vi "TXT_to_Pos_Array.vi"(11 "pointfile":path) -> (0 "errorString":string, 1 "pointIDs":string[](array[string]), 2 "pointComments":string[](array[string]), 3 "pointsXYZArray":dbl[][](array[numeric]), 4 "File Path Out":path, 5 "Number of Points":i32)   [LabVIEW 2021]
uses:
  <vilib>/Math Plots/3D Math Plots/3D Scatter/3D Scatter XCtrl/3D Scatter.xctl
  <vilib>/Math Plots/3D Math Plots/3D Plot/3D Plot Datatype/3D Plot Datatype.lvclass
  Globals/Trav_pos_global.vi
  <vilib>/Utility/file.llb/Read Delimited Spreadsheet (string).vi
  <vilib>/Math Plots/3D Math Plots/3D Scatter/3D Scatter Datatype/Public/Plot Helper (Vector).vi
  <vilib>/Math Plots/3D Math Plots/3D Scatter/3D Scatter Datatype/3D Scatter Datatype.lvclass
panel:
  out "fileRead":string[][](array[string])
  out "pointCloud":refnum<class "3D Plot Datatype.lvclass">[](xcontrol)
  # "If relative path given, prepended with path to MR file"
  # "Expects 4-row header!"
  # "Sometimes this indicator disappears..."
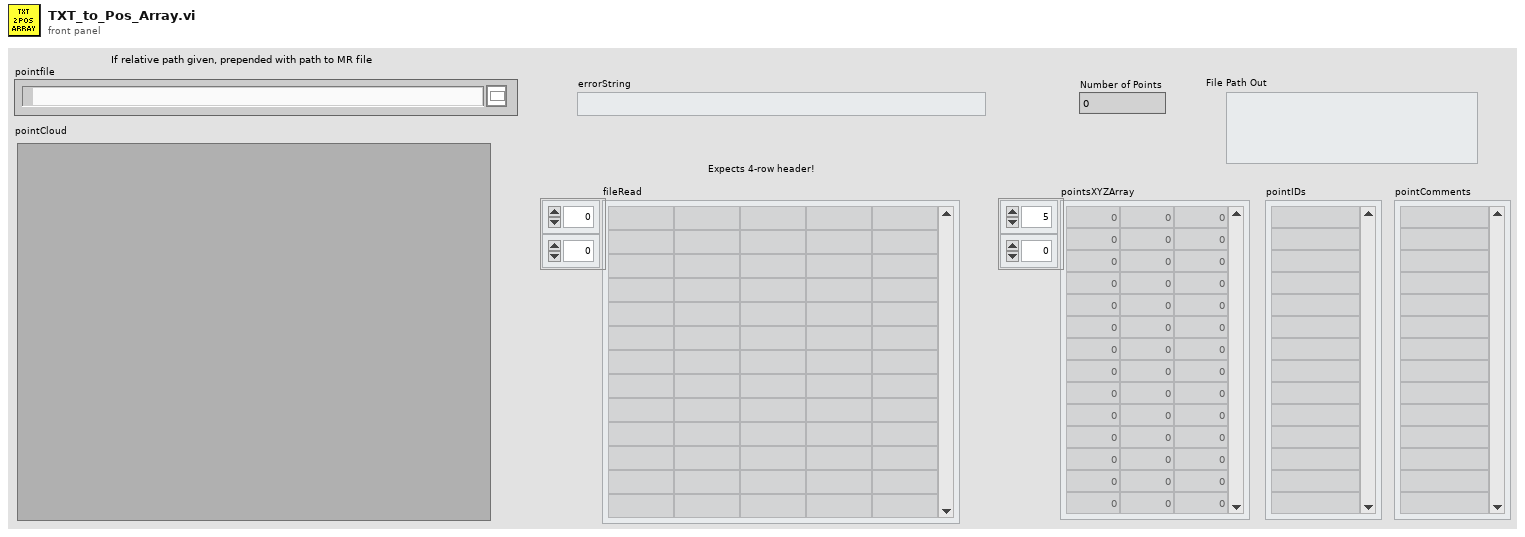
[diagram p1: front panel]
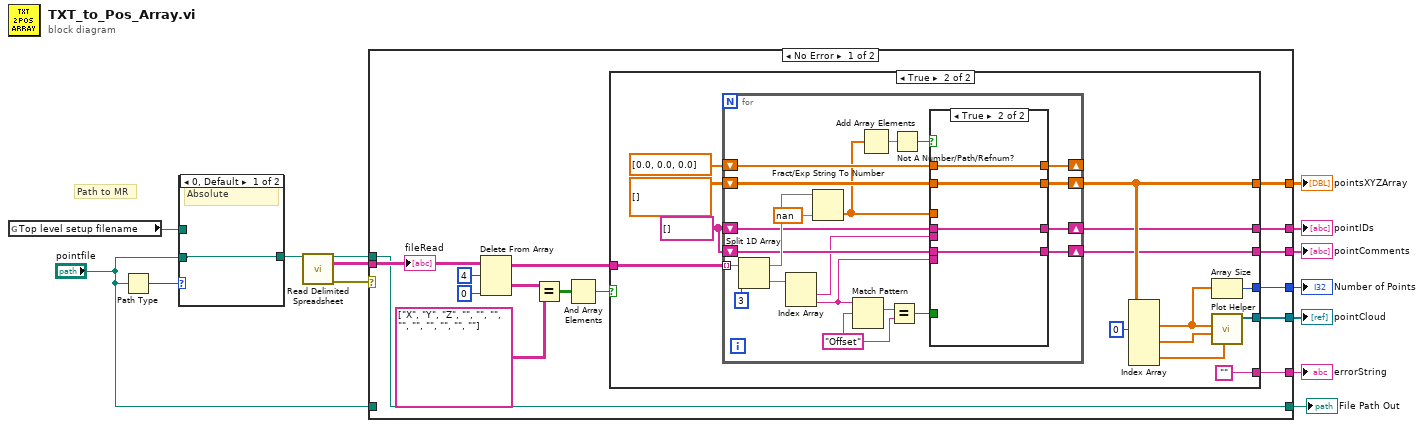
[diagram p0: block diagram]
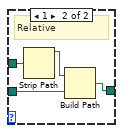
[diagram p2: hidden frame]
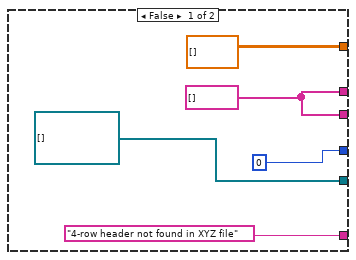
[diagram p3: hidden frame]
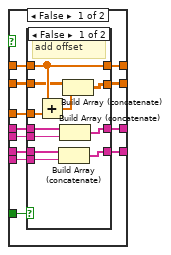
[diagram p4: hidden frame]
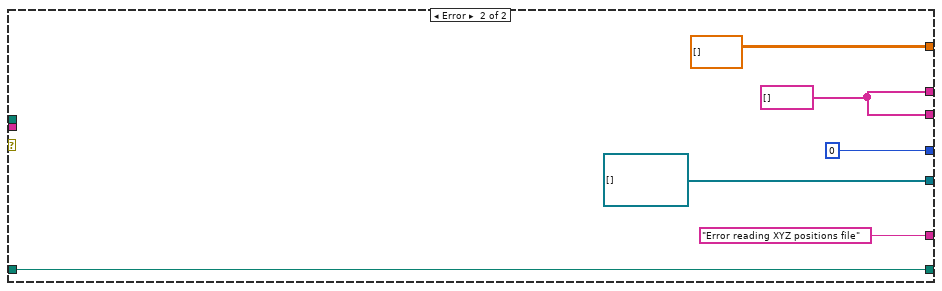
[diagram p6: hidden frame]
diagram:
  # "Path to MR"
  n1 = global read "Trav_pos_global.vi" "Top level setup filename"() -> (w6:path)
  n2 = Path Type(1:"pointfile") -> (0:w5:i16)
  n3 = case shown="0, Default" w5 {
    tunnel: w6 -> [_ w17]
    tunnel: "pointfile" -> [w15 w19]
    tunnel: [w15 w16] -> w4
    frame 0, Default {
      # "Absolute"
    }
    frame 1 {
      # "Relative"
      n4 = Strip Path(path=w17) -> (stripped path=w18:path)  [unwired: 1 out]
      n5 = Build Path(base path=w18, name or relative path=w19) -> (appended path=w16:path)
    }
  }
  n6 = call-poly <vilib>:"Read Delimited Spreadsheet.vi"("file path (dialog if empty)"=w4) -> ("new file path (Not A Path if cancelled)"=w3:path, "all rows"=w12:string[][], "error out"=w11:errorcluster)  [unwired: 9 in, 3 out]
  n7 = case shown="No Error" w11 {
    tunnel: [w34 0] -> w14
    tunnel: [w33 refnum<class "3D Plot Datatype.lvclass">[] [] ("3D Plot lvclass Array out")] -> w13
    tunnel: w12 -> [w32 _]
    tunnel: [w28 dbl[][] []] -> w9
    tunnel: [w23 "Error reading XYZ positions file"] -> w10
    tunnel: [w22 w107] -> w8
    tunnel: [w21 w107] -> w7
    tunnel: w3 -> [w20 _]
    tunnel: [w20 w106] -> w2
    tunnel: "pointfile" -> [_ w106]
    frame No Error {
      n8 = Delete From Array(array=w32, length=4, index (row)=0) -> (deleted portion=w27:string[][], array with subset deleted=w31:string[][])  [unwired: 1 in]
      n9 = Equal?(x=w27, y=string[][] [["X", "Y", "Z"], ["", "", ""], ["", "", ""], ["", "", ""]] ("deleted portion")) -> (x = y?=w25:bool[][])
      n10 = And Array Elements(Boolean array=w25) -> (logical AND=w24:bool)
      n11 = case shown="True" w24 {
        tunnel: [0 w53] -> w34
        tunnel: [refnum<class "3D Plot Datatype.lvclass">[] [] ("3D Plot lvclass Array out") w48] -> w33
        tunnel: w31 -> [_ w47]
        tunnel: [dbl[][] [] w46] -> w28
        tunnel: ["4-row header not found in XYZ file" ""] -> w23
        tunnel: [w35 w42] -> w22
        tunnel: [w35 w41] -> w21
        frame False {
          w35 = string[] []
        }
        frame True {
          w40 = string[] []
          n12 = for {
            tunnel: w47 -> [w74] mode=indexing
            shift-right: [w72] -> _
            shift-left: dbl[] [0.0, 0.0, 0.0] -> [w71]
            shift-right: [w69] -> w46
            shift-left: dbl[][] [] -> [w70]
            shift-right: [w63] -> w42
            shift-left: w40 -> [w64]
            shift-right: [w60] -> w41
            shift-left: w40 -> [w59]
            w67 = "Offset" ("element")
            n13 = Split 1D Array(array=w74, index=3 ("length")) -> (first subarray=w73:string[], second subarray=w65:string[])
            n14 = Index Array(array=w65) -> (element #1=w58:string, element #2=w61:string)  [unwired: 2 in]
            n15 = Fract/Exp String To Number(string=w73, default (0 dbl)=nan ("default (0 DBL)")) -> (number=w56:dbl[])  [unwired: 2 in, 1 out]
            n16 = Match Pattern(string=w61, regular expression=w67) -> (match substring=w68:string)  [unwired: 1 in, 3 out]
            n17 = Add Array Elements(numeric array=w56) -> (sum=w55:dbl)
            n18 = Equal?(x=w68, y=w67) -> (x = y?=w66:bool)
            n19 = Not A Number/Path/Refnum?(number/path/refnum=w55) -> (NaN/Path/Refnum?=w54:bool)
            n20 = case shown="True" w54 {
              tunnel: [w86 w105] -> w72
              tunnel: w56 -> [w85 _]
              tunnel: w71 -> [w84 w105]
              tunnel: w70 -> [w83 w104]
              tunnel: [w82 w104] -> w69
              tunnel: w66 -> [w81 _]
              tunnel: w64 -> [w80 w102]
              tunnel: [w79 w102] -> w63
              tunnel: w61 -> [w78 _]
              tunnel: [w77 w103] -> w60
              tunnel: w59 -> [w76 w103]
              tunnel: w58 -> [w75 _]
              frame False {
                n21 = case shown="False" w81 {
                  tunnel: [w96 w101] -> w86
                  tunnel: w85 -> [w97 w101]
                  tunnel: w84 -> [w96 _]
                  tunnel: w83 -> [w94 w100]
                  tunnel: [w93 w100] -> w82
                  tunnel: w78 -> [w92 _]
                  tunnel: w80 -> [w91 w99]
                  tunnel: [w90 w99] -> w79
                  tunnel: w76 -> [w88 w98]
                  tunnel: [w89 w98] -> w77
                  tunnel: w75 -> [w87 _]
                  frame False {
                    # "add offset"
                    n22 = Add(x=w96, y=w97) -> (x+y=w95:dbl[])
                    n23 = Build Array (concatenate)(w91, w92) -> (w90:string[])
                    n24 = Build Array (concatenate)(w88, w87) -> (w89:string[])
                    n25 = Build Array (concatenate)(w94, w95) -> (w93:dbl[][])
                  }
                  frame True {
                    # "store offset"
                  }
                }
              }
              frame True {
              }
            }
          }
          n26 = Index Array(array=w46, index (col) #1=0 ("disabled index (col)")) -> (element #1=w51:dbl[], element #2=w50:dbl[], element #3=w49:dbl[])  [unwired: 5 in]
          n27 = Array Size(array=w51) -> (size(s)=w53:i32)
          n28 = call-poly <vilib>:"Plot Helper.vi"("z vector"=w49, "y vector"=w50, "x vector"=w51) -> ("3D Plot lvclass Array out"=w48:refnum<class "3D Plot Datatype.lvclass">[])  [unwired: 3 in, 5 out]
        }
      }
      "fileRead" <- w32
    }
    frame Error {
      w107 = string[] []
    }
  }
  "Number of Points" <- w14
  "pointCloud" <- w13
  "pointsXYZArray" <- w9
  "errorString" <- w10
  "pointComments" <- w8
  "pointIDs" <- w7
  "File Path Out" <- w2
